vi "_078.vi"() -> ()   [LabVIEW 2024]
panel:
  out "Array 3":dbl[][](array[numeric])
  out "Array 2":dbl[][](array[numeric])
  out "max value 3":i32
  out "Array":dbl[][](array[numeric])
  out "max value 2":i32
  out "min index(es)":i32[](array[numeric])
  out "min value":i32
  out "max index(es)":i32[](array[numeric])
  out "max value":i32
  # "Fundamentals :"
  # "7~>After running this VI,what is the value displayed in the o/p ?"
  # "Nrml Approach :"
  # "Dfrnt Approach :"
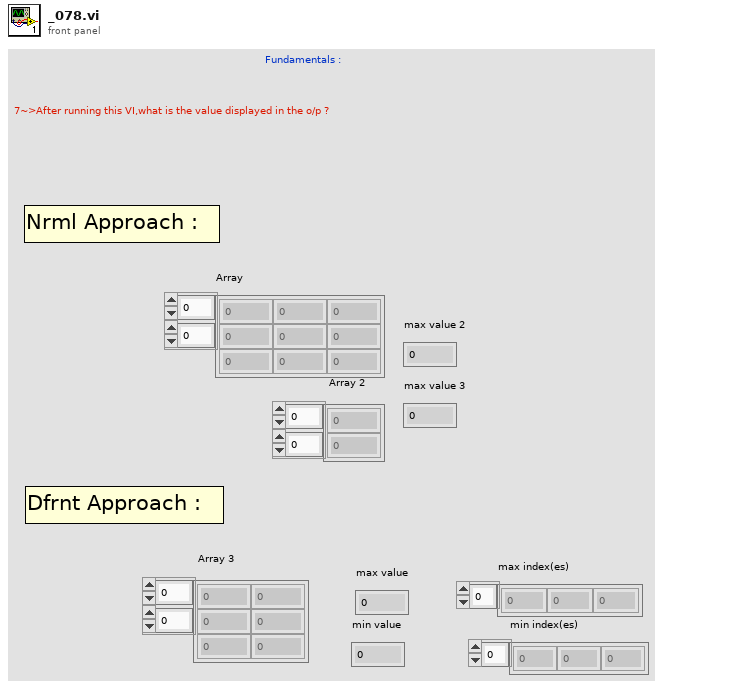
[diagram p1: front panel]
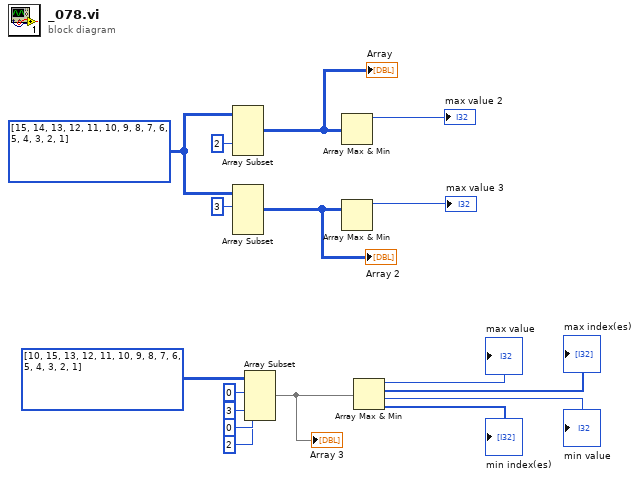
[diagram p0: block diagram]
diagram:
  w6 = i32[][] [[15, 14, 13, 12, 11], [10, 9, 8, 7, 6], [5, 4, 3, 2, 1]]
  n1 = Array Subset "Array Subset"(array=w6, index (col)=2 ("index")) -> (w7:i32[][])  [unwired: 3 in]
  "Array" <- w7
  n2 = Array Subset "Array Subset"(array=w6, index (row)=3 ("index")) -> (w3:i32[][])  [unwired: 3 in]
  "Array 2" <- w3
  n3 = Array Subset "Array Subset"(array=i32[][] [[10, 15, 13, 12, 11], [10, 9, 8, 7, 6], [5, 4, 3, 2, 1]], index (row)=0 ("index"), length (row)=3 ("length"), index (col)=0 ("index"), length (col)=2 ("length")) -> (w2:i32[][])
  "Array 3" <- w2
  n4 = Array Max & Min(array=w7) -> (max value=→"max value 2":i32)  [unwired: 3 out]
  n5 = Array Max & Min(array=w3) -> (max value=→"max value 3":i32)  [unwired: 3 out]
  n6 = Array Max & Min(array=w2) -> (max value=→"max value":i32, max index (indices)=→"max index(es)":i32[], min value=→"min value":i32, min index (indices)=→"min index(es)":i32[])
